vi "Write freq.vi"(8 "error in (no error)":errorcluster, 10 "freq":i64, 11 "Send Change Frequency MSG in":refnum<class "Send Change Frequency MSG.lvclass">) -> (0 "error out":errorcluster, 3 "Send Change Frequency MSG out":refnum<class "Send Change Frequency MSG.lvclass">)   [LabVIEW 2014, in "Controller.lvlib" / "Send Change Frequency MSG.lvclass"]
uses:
  Send Change Frequency MSG.lvclass
  Send Change Frequency MSG.lvclass/Send Change Frequency MSG.ctl
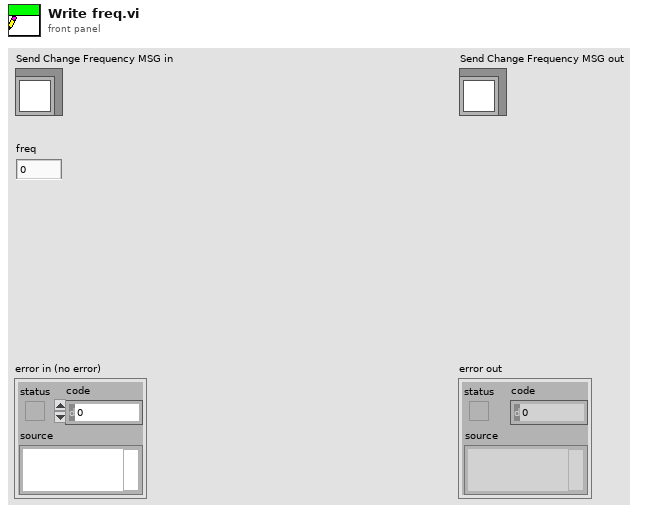
[diagram p1: front panel]
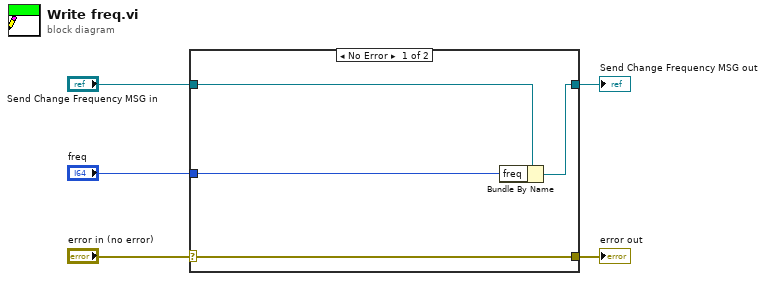
[diagram p0: block diagram]
diagram:
  n1 = case shown="No Error" "error in (no error)" {
    selector: "error in (no error)" -> [w9 w10]
    tunnel: [w9 w10] -> w4
    tunnel: [w7 w11] -> w2
    tunnel: "Send Change Frequency MSG in" -> [w8 w11]
    tunnel: "freq" -> [w6 _]
    frame No Error {
      n2 = Bundle By Name(cluster=w8, "freq"=w6) -> (w7:refnum<class "Send Change Frequency MSG.lvclass">)
    }
    frame Error {
    }
  }
  "error out" <- w4
  "Send Change Frequency MSG out" <- w2
